vi "MainLogLoop.vi"() -> ()   [LabVIEW 2014]
uses:
  <vilib>/Rock Robotics/WPI/Accelerometer/WPI_AccelerometerDevRef.ctl
  <vilib>/Rock Robotics/SystemInterfaces/Typedef/FPGA_TypedefAnalogModule.ctl
  <vilib>/Rock Robotics/WPI/Accelerometer/WPI_AccelerometerScaling.ctl
  <vilib>/Rock Robotics/WPI/Accelerometer/WPI_AccelerometerAnalogChannels.ctl
  <vilib>/Rock Robotics/SystemInterfaces/AI/FPGA_AIChannel.ctl
  <vilib>/Rock Robotics/SystemInterfaces/i2clib/i2c_bus.ctl
  <vilib>/Rock Robotics/SystemInterfaces/spilib/spi_bus.ctl
  <vilib>/Rock Robotics/WPI/Accelerometer/ADXL345 Range.ctl
  <vilib>/Rock Robotics/WPI/Accelerometer/WPI_AccelerometerADXL345 Axes.ctl
  <vilib>/Rock Robotics/WPI/SerialPort/WPI_SerialPort.ctl
  <vilib>/Rock Robotics/WPI/Accelerometer/InternalAccelerometer/WPI_AccelerometerInternalOpen.vi
panel:
  in  "AccelerometerDevRef":T1={"DevStatus"={"status"=FALSE, "code"=0, "source"=""}, "Controller"=enum."Controller 1", "Scaling"={"Gain (VoltsPerG)"=0.0, "Center Voltage"=0.0}, "Analog Channels"={"X-Axis"=enum."Invalid", "Y-Axis"=enum."Invalid", "Z-Axis"=enum."Invalid"}, "I2C Bus"=enum."Invalid", "SPI Bus"=enum."Invalid", "Accel Range"=0, "ADXL345 Axes"={"X-Axis"=FALSE, "Y-Axis"=FALSE, "Z-Axis"=FALSE}, "Handle"=0, "Device Address"=0, "Accel Type"=enum."Analog"} {"Device Address" format="%.0x"; "Accel Range" items=["+/- 2 g", "+/- 4 g", "+/- 8 g", "+/- 16 g"]}
  out "error out":errorcluster
  in  "error in (no error)":errorcluster
  # "ADXL345"
  # "Analog"
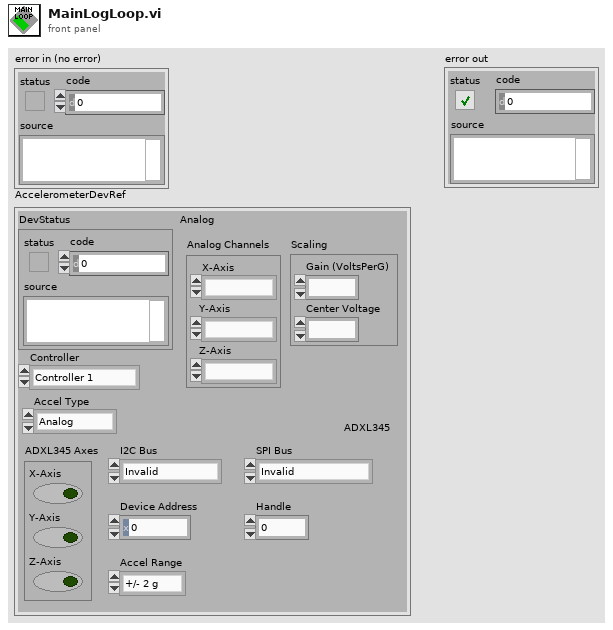
[diagram p1: front panel]
types:
  T1 = typedef "WPI_AccelerometerDevRef.ctl" = cluster{"DevStatus":errorcluster, "Controller":T2, "Scaling":T3, "Analog Channels":T4, "I2C Bus":T6, "SPI Bus":T7, "Accel Range":T8, "ADXL345 Axes":T9, "Handle":i32, "Device Address":u8, "Accel Type":enum16{"Analog", "ADXL345 I2C", "ADXL345 SPI", "Internal"}}
  T2 = typedef "FPGA_TypedefAnalogModule.ctl" = enum16{"Controller 1"}
  T3 = typedef "WPI_AccelerometerScaling.ctl" = cluster{"Gain (VoltsPerG)":dbl, "Center Voltage":dbl}
  T4 = typedef "WPI_AccelerometerAnalogChannels.ctl" = cluster{"X-Axis":T5, "Y-Axis":T5, "Z-Axis":T5}
  T5 = typedef "FPGA_AIChannel.ctl" = enum8{"AI 0", "AI 1", "AI 2", "AI 3", "AI MXP 0", "AI MXP 1", "AI MXP 2", "AI MXP 3", "Invalid"}
  T6 = typedef "i2c_bus.ctl" = enum16{"I2C On-Board", "I2C MXP", "Invalid"}
  T7 = typedef "spi_bus.ctl" = enum16{"SPI On-Board, CS0", "SPI On-Board, CS1", "SPI On-Board, CS2", "SPI On-Board, CS3", "SPI MXP", "Invalid"}
  T8 = typedef "ADXL345 Range.ctl" = u8
  T9 = typedef "WPI_AccelerometerADXL345 Axes.ctl" = cluster{"X-Axis":bool, "Y-Axis":bool, "Z-Axis":bool}
  T10 = typedef "WPI_SerialPort.ctl" = enum16{"Onboard RS-232", "MXP TTL"}
  T11 = typedef "WPI_SerialPortRef.ctl" = cluster{"DevStatus":errorcluster, "Serial Port Name":refnum<visa-resource-name>}
  T12 = cluster{"X-Axis":dbl, "Y-Axis":dbl, "Z-Axis":dbl}
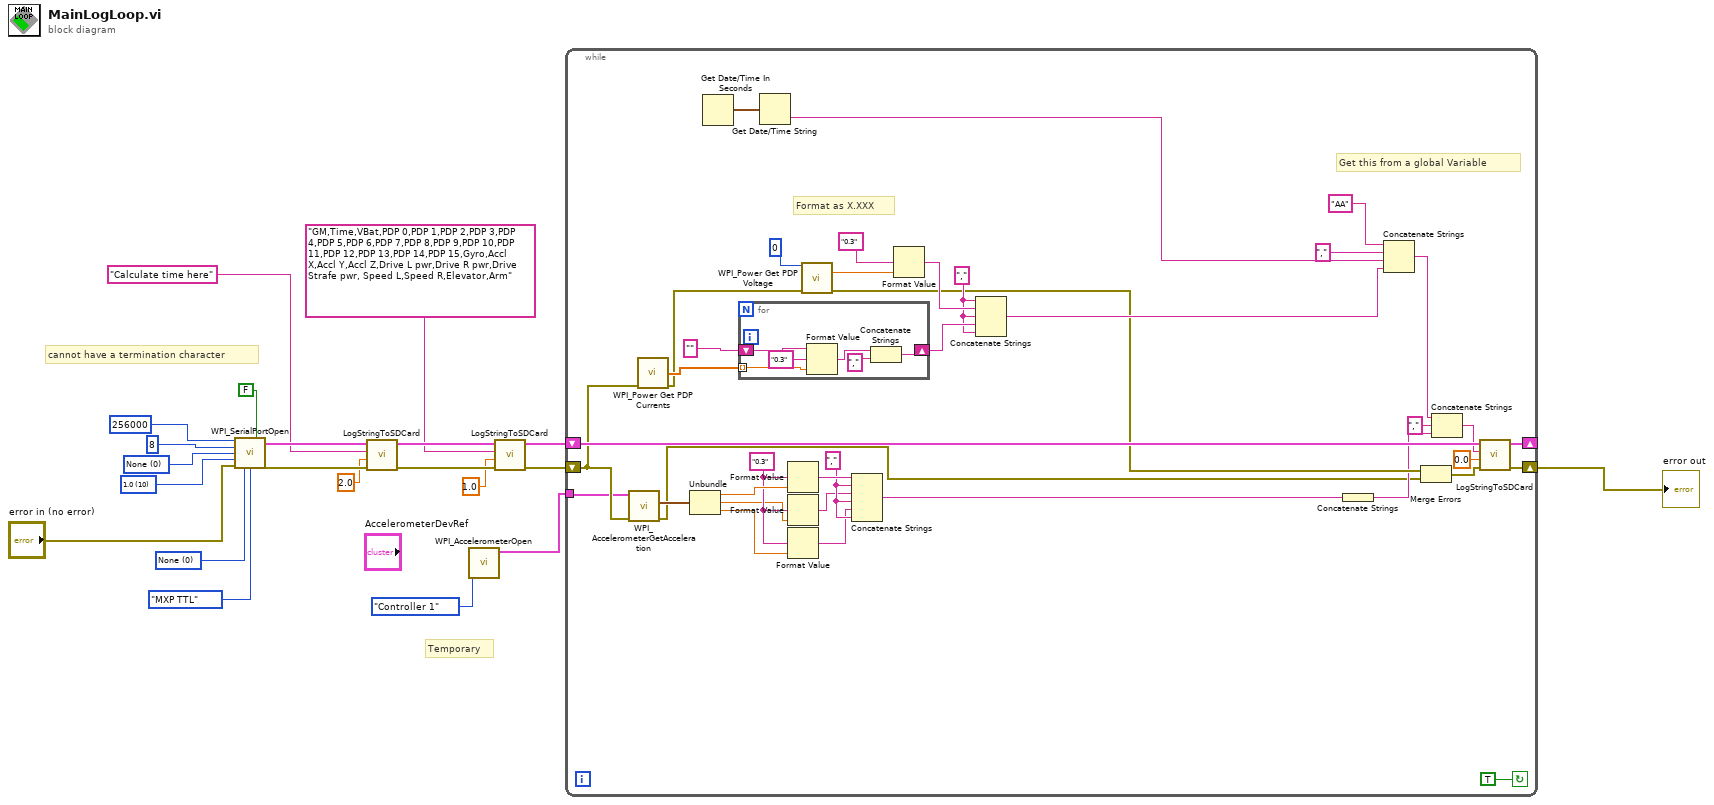
[diagram p0: block diagram]
diagram:
  w17 = u16 0 items=["None", "XON/XOFF", "RTS/CTS", "XON/XOFF & RTS/CTS", "DTR/DSR", "XON/XOFF & DTR/DSR"] ("Flow Control")
  w18 = u16 10 items=["1.0"=10, "1.5"=15, "2.0"=20] ("Stop Bits")
  w19 = u16 0 items=["None", "Odd", "Even", "Mark", "Space"] ("Parity")
  # "Temporary"
  # "cannot have a termination character"
  n1 = call <vilib>:"WPI_SerialPortOpen.vi"("Baud Rate"=u32 256000, "Enable Termination Char? (T)"=FALSE, "Data Bits"=u16 8, "Parity"=w19, "Stop Bits"=w18, "error in (no error)"="error in (no error)", "Flow Control"=w17, "Serial Port"=WPI_SerialPort."MXP TTL") -> ("SerialPortRef"=w13:T11, "error out"=w12:errorcluster)  [unwired: 6 in]
  n2 = call "LogStringToSDCard.vi"("error in (no error)"=w12, "Log Type"=2.0, "Log string"="Calculate time here", "SerialPortRef"=w13) -> ("error out"=w10:errorcluster, "SerialPortRef out"=w11:T11)  [unwired: 4 in]
  n3 = call-poly <vilib>:"WPI_AccelerometerOpen.vi"("Controller"=FPGA_TypedefAnalogModule."Controller 1") -> ("AccelerometerDevRef"=w2:T1)  [unwired: 9 in, 1 out]
  n4 = call "LogStringToSDCard.vi"("error in (no error)"=w10, "Log Type"=1.0, "Log string"="GM,Time,VBat,PDP 0,PDP 1,PDP 2,PDP 3,PDP 4,PDP 5,PDP 6,PDP 7,PDP 8,PDP 9,PDP 10,PDP 11,PDP 12,PDP 13,PDP 14,PDP 15,Gyro,Accl X,Accl Y,Accl Z,Drive L pwr,Drive R pwr,Drive Strafe pwr, Speed L,Speed R,Elevator,Arm", "SerialPortRef"=w11) -> ("error out"=w8:errorcluster, "SerialPortRef out"=w7:T11)  [unwired: 4 in]
  n5 = while {
    shift-right: [w57] -> w3
    shift-left: w8 -> [w37]
    shift-right: [w58] -> _
    shift-left: w7 -> [w59]
    tunnel: w2 -> [w34]
    stop <- TRUE continue-if-true
    w30 = ","
    w27 = "0.3" ("format string")
    w46 = "," ("string")
    # "Get this from a global Variable"
    # "Format as X.XXX"
    n6 = call <vilib>:"WPI_AccelerometerGetAcceleration.vi"("error in"=w37, "AccelerometerDevRef"=w34) -> ("error out"=w22:errorcluster, "Accelerations"=w33:T12)  [unwired: 7 in, 1 out]
    n7 = call <vilib>:"WPI_Power Get PDP Currents.vi"("error in"=w37) -> ("all currents (A)"=w52:dbl[], "error out"=w49:errorcluster)  [unwired: 12 in, 1 out]
    n8 = Unbundle(w33) -> ("X-Axis"=w31:dbl, "Y-Axis"=w25:dbl, "Z-Axis"=w26:dbl)
    n9 = Get Date/Time In Seconds() -> (seconds since 1Jan1904=w48:timestamp)
    n10 = for {
      tunnel: w52 -> [w60] mode=indexing
      shift-right: [w63] -> w50
      shift-left: "" -> [w65]
      n11 = Format Value(string ("")=w65, format string="0.3", value (0)=w60) -> (output string=w62:string)
      n12 = Concatenate Strings(w62, ",") -> (w63:string)
    }
    n13 = Get Date/Time String(seconds (now)=w48) -> (time string=w47:string)  [unwired: 2 in, 1 out]
    n14 = Format Value(format string=w27, value (0)=w31) -> (output string=w32:string)  [unwired: 1 in]
    n15 = Format Value(format string=w27, value (0)=w25) -> (output string=w29:string)  [unwired: 1 in]
    n16 = Format Value(format string=w27, value (0)=w26) -> (output string=w28:string)  [unwired: 1 in]
    n17 = call <vilib>:"WPI_Power Get PDP Voltage.vi"("Power Distribution Panel (0)"=u8 0, "error in"=w49) -> ("voltage (V)"=w56:dbl, "error out"=w35:errorcluster)  [unwired: 12 in]
    n18 = Concatenate Strings(w32, w30, w29, w30, w28, w30) -> (w24:string)
    n19 = Format Value(format string="0.3", value (0)=w56) -> (output string=w53:string)  [unwired: 1 in]
    n20 = Concatenate Strings(w46, w53, w46, w50, w46) -> (w45:string)
    n21 = Concatenate Strings(w24) -> (w23:string)
    n22 = Concatenate Strings("AA" ("string"), "," ("string"), w47, w45) -> (w41:string)
    n23 = Merge Errors(w35, w22) -> (w36:errorcluster)
    n24 = Concatenate Strings(w41, "," ("string"), w23) -> (w40:string)
    n25 = call "LogStringToSDCard.vi"("error in (no error)"=w36, "Log Type"=0.0, "Log string"=w40, "SerialPortRef"=w59) -> ("error out"=w57:errorcluster, "SerialPortRef out"=w58:T11)  [unwired: 4 in]
  }
  "error out" <- w3
